vi "Table_to_Sample_positions.vi"(1 "Table":string[][](table)) -> (0 "Sample Positions array":T1[](array[typedef]) {"Z" format="%.1f"; "Y" format="%.1f"; "X" format="%.1f"; "SAMPLE NO." min=1 max=40 step=1})   [LabVIEW 2010]
uses:
  Controls/Sample_pos.ctl
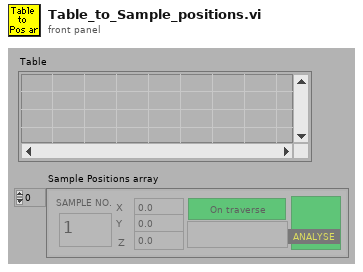
[diagram p1: front panel]
types:
  T1 = typedef "Sample_pos.ctl" = cluster{"SAMPLE NO.":i32, "X":dbl, "Y":dbl, "Z":dbl, "On trav":bool, "Analyse?":bool, "Notes":string}
  T2 = cluster{"[0]":dbl, "[1]":dbl, "[2]":dbl, "[3]":dbl}
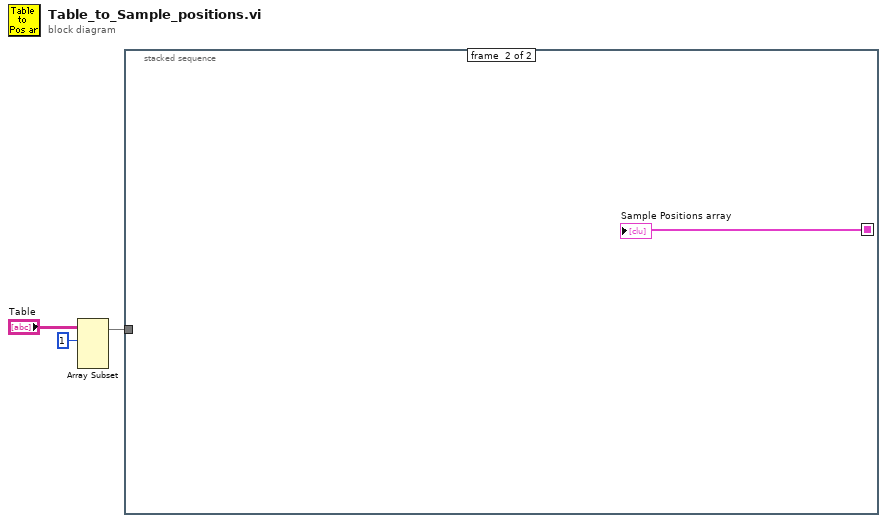
[diagram p0: block diagram]
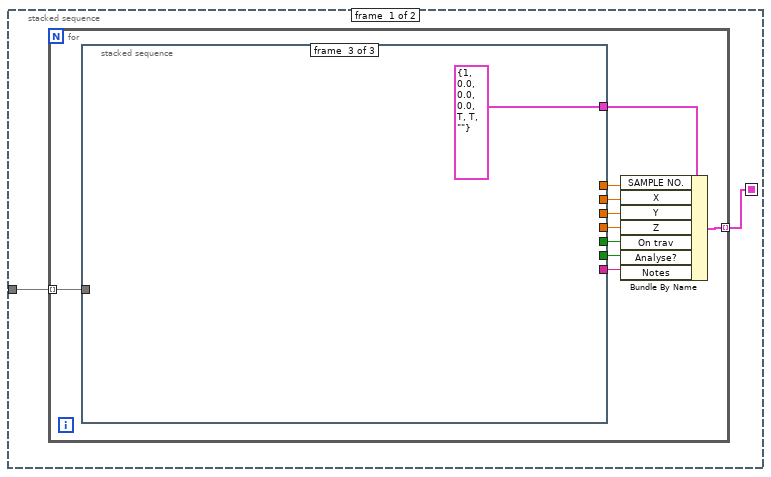
[diagram p2: hidden frame]
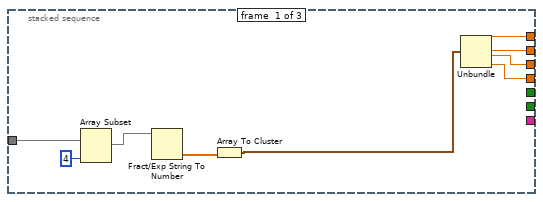
[diagram p3: hidden frame]
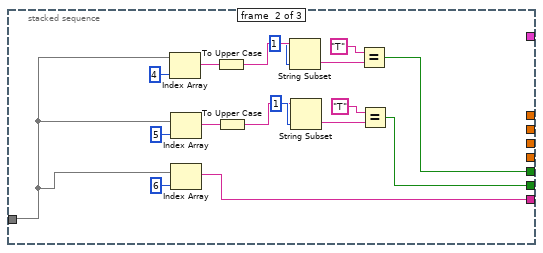
[diagram p4: hidden frame]
diagram:
  n1 = Array Subset(array="Table", index (row)=1) -> (w2:string[][])  [unwired: 3 in]
  n2 = stacked-sequence {
    seq-local: [w4 _] -> [_ w43]
    tunnel: w2 -> [w5 _]
    frame #0 {
      n3 = for {
        tunnel: w5 -> [w14] mode=indexing
        tunnel: [w6] -> w4 mode=indexing
        n4 = stacked-sequence {
          tunnel: [_ _ T1 {"SAMPLE NO."=1, "X"=0.0, "Y"=0.0, "Z"=0.0, "On trav"=TRUE, "Analyse?"=TRUE, "Notes"=""}] -> w15
          tunnel: w14 -> [w16 w28 _]
          tunnel: [w20 _ _] -> w13
          tunnel: [w19 _ _] -> w12
          tunnel: [w18 _ _] -> w11
          tunnel: [w17 _ _] -> w10
          tunnel: [_ w27 _] -> w9
          tunnel: [_ w26 _] -> w8
          tunnel: [_ w25 _] -> w7
          frame #0 {
            n5 = Array Subset(array=w16, length=4) -> (w23:string[])  [unwired: 1 in]
            n6 = Fract/Exp String To Number(string=w23) -> (number=w22:dbl[])  [unwired: 3 in, 1 out]
            n7 = Array To Cluster(array=w22) -> (cluster=w21:T2)
            n8 = Unbundle(w21) -> ("[0]"=w20:dbl, "[1]"=w19:dbl, "[2]"=w18:dbl, "[3]"=w17:dbl)
          }
          frame #1 {
            n9 = Index Array(array=w28, index=4) -> (element=w37:string)
            n10 = Index Array(array=w28, index=5) -> (element=w34:string)
            n11 = Index Array(array=w28, index=6) -> (element=w27:string)
            n12 = To Upper Case(1:w37) -> (0:w39:string)
            n13 = To Upper Case(1:w34) -> (0:w32:string)
            n14 = String Subset(string=w39, length (rest)=1 ("length")) -> (substring=w40:string)  [unwired: 1 in]
            n15 = String Subset(string=w32, length (rest)=1 ("length")) -> (substring=w31:string)  [unwired: 1 in]
            n16 = Equal?(x="T", y=w40) -> (x = y?=w25:bool)
            n17 = Equal?(x="T", y=w31) -> (x = y?=w26:bool)
          }
          frame #2 {
          }
        }
        n18 = Bundle By Name(cluster=w15, "SAMPLE NO."=w13, "X"=w12, "Y"=w11, "Z"=w10, "On trav"=w7, "Analyse?"=w8, "Notes"=w9) -> (w6:T1)
      }
    }
    frame #1 {
      "Sample Positions array" <- w43
    }
  }
